vi "ledswitharrays.vi"() -> ()   [LabVIEW 2015]
panel:
  out "Led 11":bool
  out "Led 10":bool
  out "Led 9":bool
  out "subarray":bool[](array[boolean])
  in  "stop":bool
  out "Led 8":bool
  out "Led 7":bool
  out "Led 6":bool
  out "Led 5":bool
  out "Led 4":bool
  out "Led 3":bool
  out "Led 2":bool
  out "Led 1":bool
  in  "Longitud de \nla secuencia":i32
  in  "Array":bool[][](array[boolean])
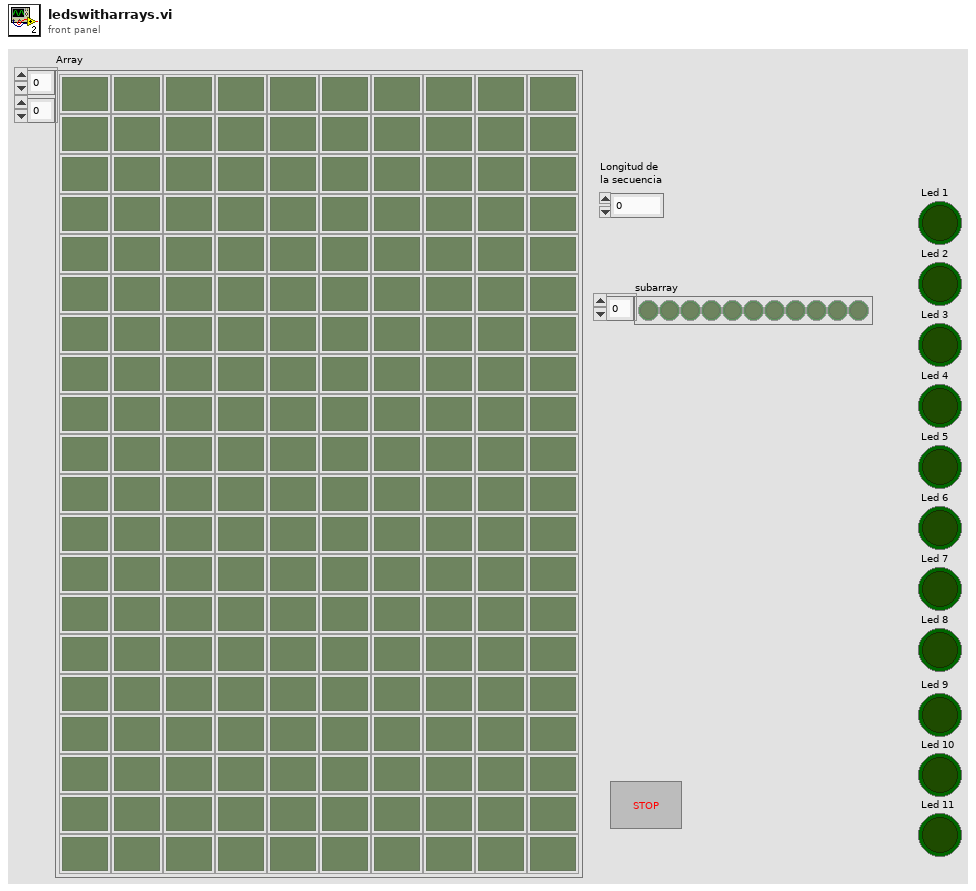
[diagram p1: front panel]
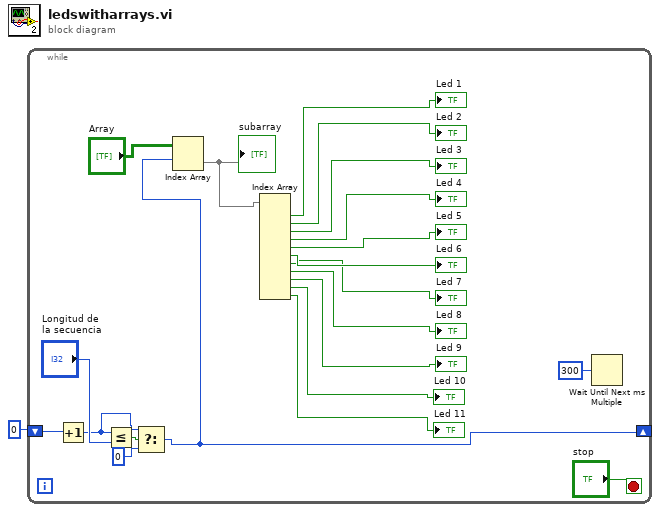
[diagram p0: block diagram]
diagram:
  n1 = while {
    shift-right: [w3] -> _
    shift-left: 0 -> [w8]
    stop <- "stop" stop-if-true
    n2 = Increment(x=w8) -> (x+1=w5:i32)
    n3 = Less Or Equal?(x=w5, y="Longitud de \nla secuencia") -> (x <= y?=w6:bool)
    n4 = Select(t=w5, s=w6, f=0) -> (s? t:f=w3:i32)
    n5 = Index Array(array="Array", index (row)=w3) -> (element=w20:bool[])  [unwired: 1 in]
    "subarray" <- w20
    n6 = Index Array(array=w20) -> (element #1=→"Led 1":bool, element #2=→"Led 2":bool, element #3=→"Led 3":bool, element #4=→"Led 4":bool, element #5=→"Led 5":bool, element #6=→"Led 6":bool, element #7=→"Led 7":bool, element #8=→"Led 8":bool, element #9=→"Led 9":bool, element #10=→"Led 10":bool, element #11=→"Led 11":bool)  [unwired: 11 in]
    n7 = Wait Until Next ms Multiple(millisecond multiple=u32 300) -> ()  [unwired: 1 out]
  }
